vi "MAC Address Fetcher_2011 SP1.vi"(8 "error in (no error)":errorcluster, 11 "Search all adapters?":bool) -> (0 "error out":errorcluster, 1 "element":string, 2 "index of element":i32, 3 "MAC Addresses":string[](array[string]))   [LabVIEW 2017]
doc: "This VI calls a Windows shell command that fetches details of the installed Network Interface Cards. It then searches for valid Physical (MAC) Addresses and populates an array. If \"All adapters\" is set to True, then the whole array will be output. otherwise, only the first element will be output, which should correspond to the primary ethernet adapter."
panel:
  out "Shell Output":string
  # "Network card MAC Address Fetcher"
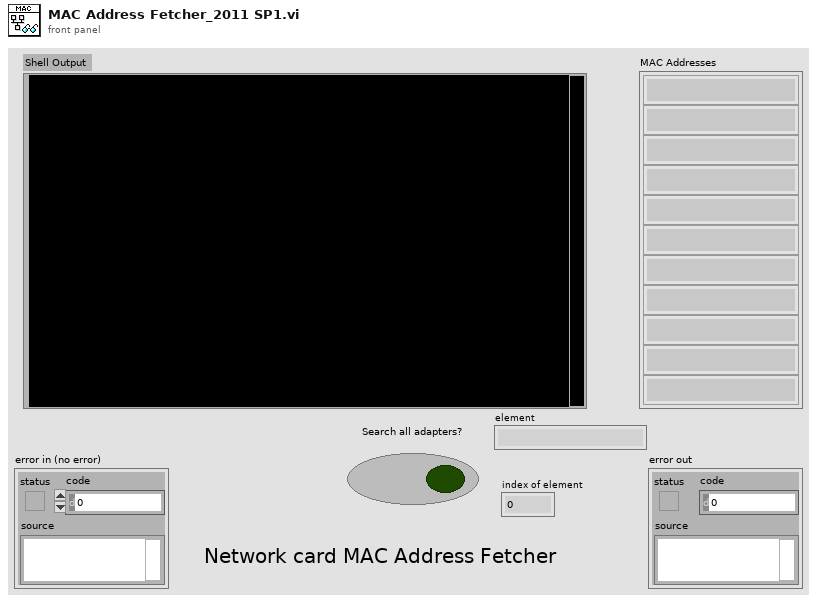
[diagram p1: front panel]
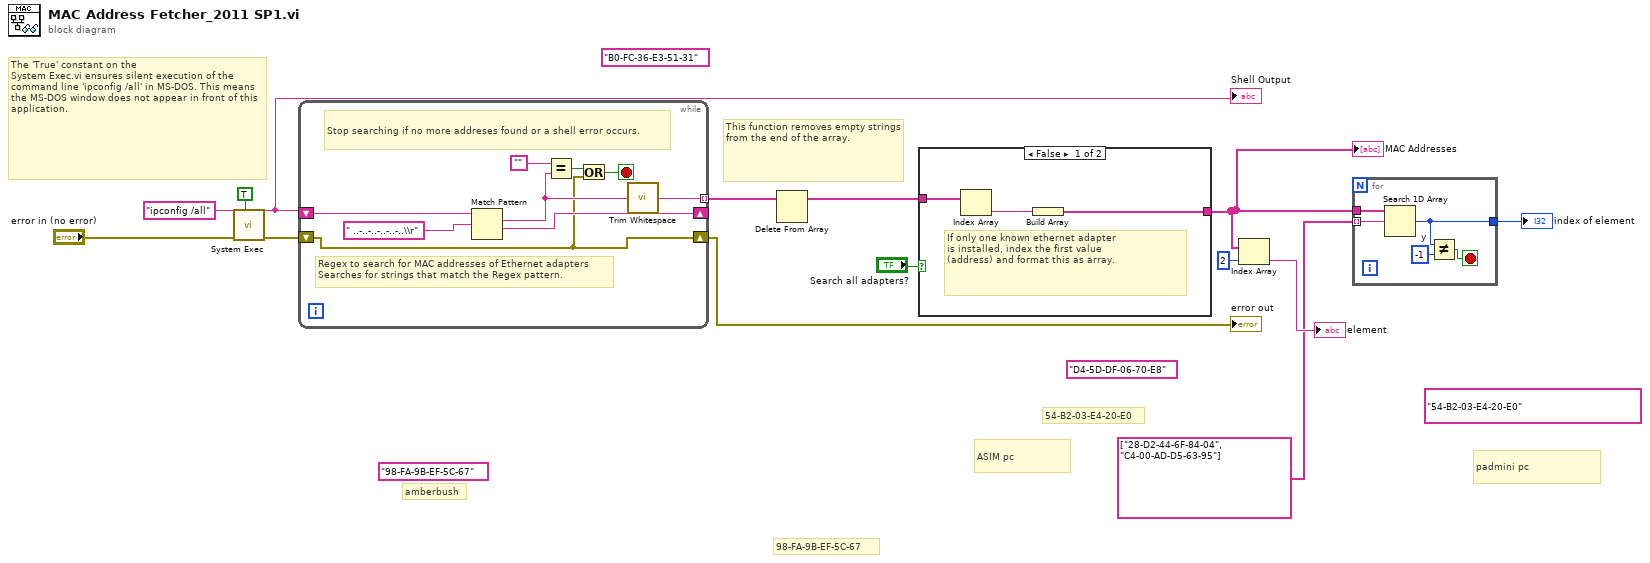
[diagram p0: block diagram]
diagram:
  (unwired) "98-FA-9B-EF-5C-67" ("element")
  (unwired) "D4-5D-DF-06-70-E8" ("element")
  (unwired) "54-B2-03-E4-20-E0" ("element")
  (unwired) "B0-FC-36-E3-51-31" ("element")
  # "ASIM pc"
  # "54-B2-03-E4-20-E0"
  # "amberbush"
  # "98-FA-9B-EF-5C-67"
  # "padmini pc"
  # "The 'True' constant on the \nSystem Exec.vi ensures silent execution of the command line 'ipconfig /all' in MS-DOS. This means the MS-DOS window does not appear in front of this application."
  # "This function removes empty strings from the end of the array."
  n1 = call <vilib>:"System Exec.vi"("run minimized? (F)"=TRUE, "error in (no error)"="error in (no error)", "command line"="ipconfig /all") -> ("error out"=w9:errorcluster, "standard output"=w12:string)  [unwired: 5 in, 2 out]
  "Shell Output" <- w12
  n2 = while {
    shift-right: [w21] -> _
    shift-left: w12 -> [w22]
    tunnel: [w15] -> w11 mode=indexing
    shift-right: [w16] -> w8
    shift-left: w9 -> [w16]
    stop <- w17 stop-if-true
    # "Stop searching if no more addreses found or a shell error occurs."
    # "Regex to search for MAC addresses of Ethernet adapters\nSearches for strings that match the Regex pattern."
    n3 = Match Pattern(string=w22, regular expression=" ..-..-..-..-..-..\\r") -> (match substring=w20:string, after substring=w21:string)  [unwired: 1 in, 2 out]
    n4 = Equal?(x="", y=w20) -> (x = y?=w18:bool)
    n5 = Or(x=w18, y=w16) -> (x .or. y?=w17:bool)
    n6 = call <vilib>:"Trim Whitespace.vi"("string"=w20) -> ("trimmed string"=w15:string)  [unwired: 1 in]
  }
  "error out" <- w8
  n7 = Delete From Array "Delete From Array"(array=w11) -> (array with subset deleted=w6:string[])  [unwired: 2 in, 1 out]
  n8 = case shown="False" "Search all adapters?" {
    tunnel: w6 -> [w26 w27]
    tunnel: [w24 w27] -> w5
    frame False {
      # "If only one known ethernet adapter \nis installed, index the first value \n(address) and format this as array."
      n9 = Index Array "Index Array"(array=w26) -> (element=w25:string)  [unwired: 1 in]
      n10 = Build Array "Build Array"(w25) -> (w24:string[])
    }
    frame True {
      # "Otherwise, output all addresses"
    }
  }
  "MAC Addresses" <- w5
  n11 = Index Array(array=w5, index=2) -> (element=→"element":string)
  n12 = for {
    tunnel: w5 -> [w32]
    tunnel: [w30] -> w3
    tunnel: string[] ["28-D2-44-6F-84-04", "C4-00-AD-D5-63-95"] ("element") -> [w31] mode=indexing
    stop <- w28 stop-if-true
    w29 = -1  # y
    n13 = Search 1D Array(1D array=w32, element=w31) -> (index of element=w30:i32)  [unwired: 1 in]
    n14 = Not Equal?(x=w30, y=w29) -> (x != y?=w28:bool)
  }
  "index of element" <- w3
